vi "provide_note_book_info.vi"(8 "error in (no error)":errorcluster, 10 "notebook string in":string, 11 "GenericPlugin in":refnum<class "ImagingModeDL100901FlexTrajectory.lvclass">) -> (0 "error out":errorcluster, 2 "notebook string out":string, 3 "GenericPlugin out":refnum<class "ImagingModeDL100901FlexTrajectory.lvclass">)   [LabVIEW 2010, in "ImagingModeDL100901FlexTrajectory.lvclass"]
uses:
  ImagingModeDL100901FlexTrajectory.lvclass
  ImagingModeDL100901FlexTrajectory.lvclass/ImagingModeDL100901FlexTrajectory.ctl
  common/classes/ErrorController/ErrorController/class_data.vi
  common/classes/ErrorController/ErrorController/ErrorController.lvclass
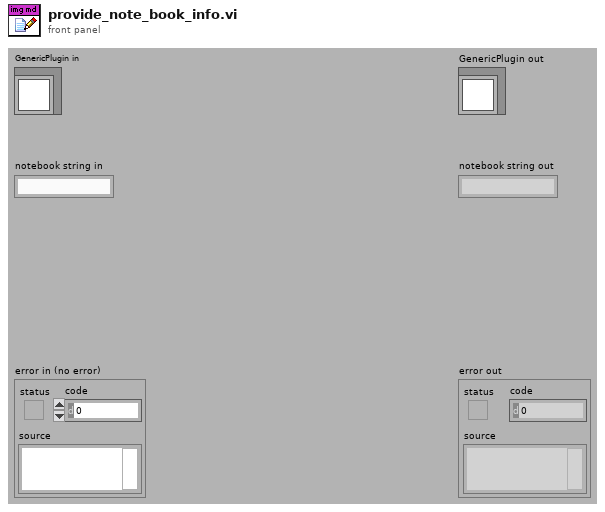
[diagram p1: front panel]
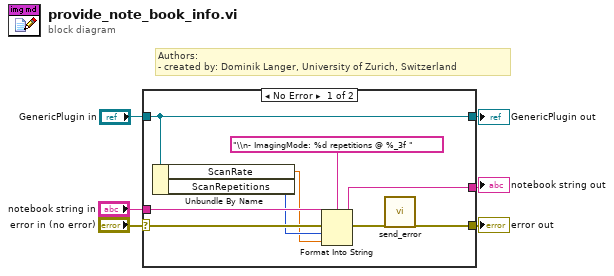
[diagram p0: block diagram]
diagram:
  # "Authors: \n- created by: Dominik Langer, University of Zurich, Switzerland"
  n1 = case shown="No Error" "error in (no error)" {
    selector: "error in (no error)" -> [w12 w18]
    tunnel: "notebook string in" -> [w13 w16]
    tunnel: "GenericPlugin in" -> [w14 w17]
    tunnel: [w15 w18] -> w6
    tunnel: [w14 w17] -> w5
    tunnel: [w8 w16] -> w1
    frame No Error {
      n2 = Unbundle By Name(w14) -> ("ScanRate"=w10:dbl[unit], "ScanRepetitions"=w11:i32)
      n3 = Format Into String(format string="\\n- ImagingMode: %d repetitions @ %_3f ", initial string=w13, error in=w12, w11, w10) -> (resulting string=w8:string, error out=w9:errorcluster)
      n4 = call "send_error.vi"("error in (no error)"=w9) -> ("error out"=w15:errorcluster)  [unwired: 10 in]
    }
    frame Error {
    }
  }
  "error out" <- w6
  "GenericPlugin out" <- w5
  "notebook string out" <- w1
